vi "Enqueue_Queue_Polymorphic.vi"   [LabVIEW 2014, in "Queue_Library.lvlib"]
uses:
  Queue_Library.lvlib
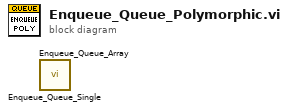
[diagram p0: block diagram]
diagram:
  n1 = call "Enqueue_Queue_Single.vi"() -> ()  [unwired: 10 in, 2 out]
  n2 = call "Enqueue_Queue_Array.vi"() -> ()  [unwired: 10 in, 2 out]
